vi "Set CD Item Property Value.vi"(8 "error in (no error)":errorcluster, 10 "CD Item Ref in":u64, 11 "Parameter in":refnum<class "Parameter.lvclass">) -> (0 "error out":errorcluster, 3 "Parameter out":refnum<class "Parameter.lvclass">)   [LabVIEW 2019, in "CD Parameter Manager API.lvlib" / "Parameter.lvclass"]
uses:
  Parameter.lvclass
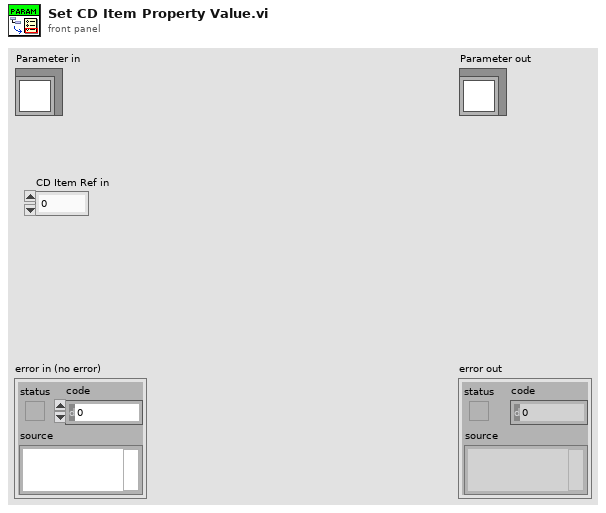
[diagram p1: front panel]
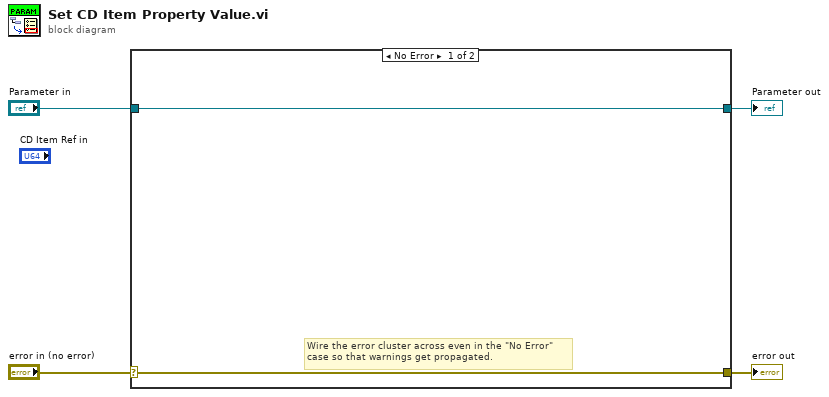
[diagram p0: block diagram]
diagram:
  n1 = case shown="No Error" "error in (no error)" {
    selector: "error in (no error)" -> [w5 w8]
    tunnel: [w5 w8] -> w3
    tunnel: [w6 w7] -> w1
    tunnel: "Parameter in" -> [w6 w7]
    frame No Error {
      # "Wire the error cluster across even in the \"No Error\"\ncase so that warnings get propagated."
    }
    frame Error {
    }
  }
  "error out" <- w3
  "Parameter out" <- w1
